vi "PPR_DRIVE_SET_GYRO.vi"(11 "Gyro Heading Radians":dbl) -> ()   [LabVIEW 2019]
uses:
  PPR_DRIVE_GLOBALS.vi
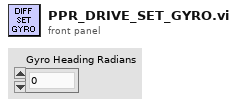
[diagram p1: front panel]
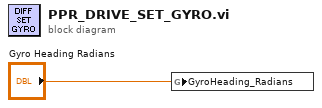
[diagram p0: block diagram]
diagram:
  n1 = global write "PPR_DRIVE_GLOBALS.vi" "GyroHeading_Radians"("Gyro Heading Radians") -> ()
